vi "Create Plugins.vi"(8 "error in (no error)":errorcluster, 9 "async plugins tag":string, 10 "inline plugins tag":string, 11 "Application Data In":T1={"Item Tree Control"=refnum, "Top-Level VI"=refnum, "menu reference"=refnum, "queue"=refnum, "Stop Pointer"=refnum, "Buffer Variant"=variant, "server ID"=refnum, "framework tag"="", "Values"=refnum, "Hex"=refnum, "ASCII"=refnum, "lines visible"=0, "values padding"=0, "current buffer data"={"decimation"=0, "avg bandwidth"=0.0, "channels"=[], "byte order"=enum."little-endian", "buffer descriptor"={"buffer type"=enum."Engine", "plugin id"=0, "group id"=0, "transfer id"=0, "offset"=0, "length"=0}, "values channels"={"index"=0, "count"=0, "engine offset"=0}, "select start offset"=18446744073709551615, "select end offset"=0, "channel index"=-1}, "Framework Configuration"=refnum} {"current buffer data"."channels"."configuration"."string offset" format="%d bytes"; "current buffer data"."avg bandwidth" format="%.0g bytes"}) -> (0 "error out":errorcluster, 2 "avg bandwidth":dbl, 3 "Application Data out":T1={"Item Tree Control"=refnum, "Top-Level VI"=refnum, "menu reference"=refnum, "queue"=refnum, "Stop Pointer"=refnum, "Buffer Variant"=variant, "server ID"=refnum, "framework tag"="", "Values"=refnum, "Hex"=refnum, "ASCII"=refnum, "lines visible"=0, "values padding"=0, "current buffer data"={"decimation"=0, "avg bandwidth"=0.0, "channels"=[], "byte order"=enum."little-endian", "buffer descriptor"={"buffer type"=enum."Engine", "plugin id"=0, "group id"=0, "transfer id"=0, "offset"=0, "length"=0}, "values channels"={"index"=0, "count"=0, "engine offset"=0}, "select start offset"=18446744073709551615, "select end offset"=0, "channel index"=-1}, "Framework Configuration"=refnum} {"current buffer data"."channels"."configuration"."string offset" format="%d bytes"; "current buffer data"."avg bandwidth" format="%.0g bytes"})   [LabVIEW 2020, in "DSF Core.lvlib"]
uses:
  DSF Core.lvlib
  Buffer Reader/Buffer Data.ctl
  Typedefs/DSF Data Type.ctl
  Typedefs/DSF Byte Order.ctl
  Typedefs/DSF Settings Info.ctl
  Typedefs/DSF Buffer Type.ctl
  Classes/Thread/Data Server/DSF Buffer Subset Descriptor.ctl
  Main VI/Values Channels.ctl
  Typedefs/Core Channel Configuration.ctl
  Classes/Configuration/Core/Channel/Channel Configuration.lvclass
  Classes/Configuration/Core/Framework/Framework Configuration.lvclass
  Classes/Configuration/Core/Plugin/Plugin Configuration.lvclass
  Classes/Configuration/Core/Transfer/Channel Configuration.ctl
  Classes/Configuration/Core/Transfer/Transfer Configuration.lvclass
  Main VI/Application Data.ctl
  <vilib>/NI/Memory Manager/Classes/Pointer/Pointer.lvclass
  Buffer Reader/Queue Data.ctl
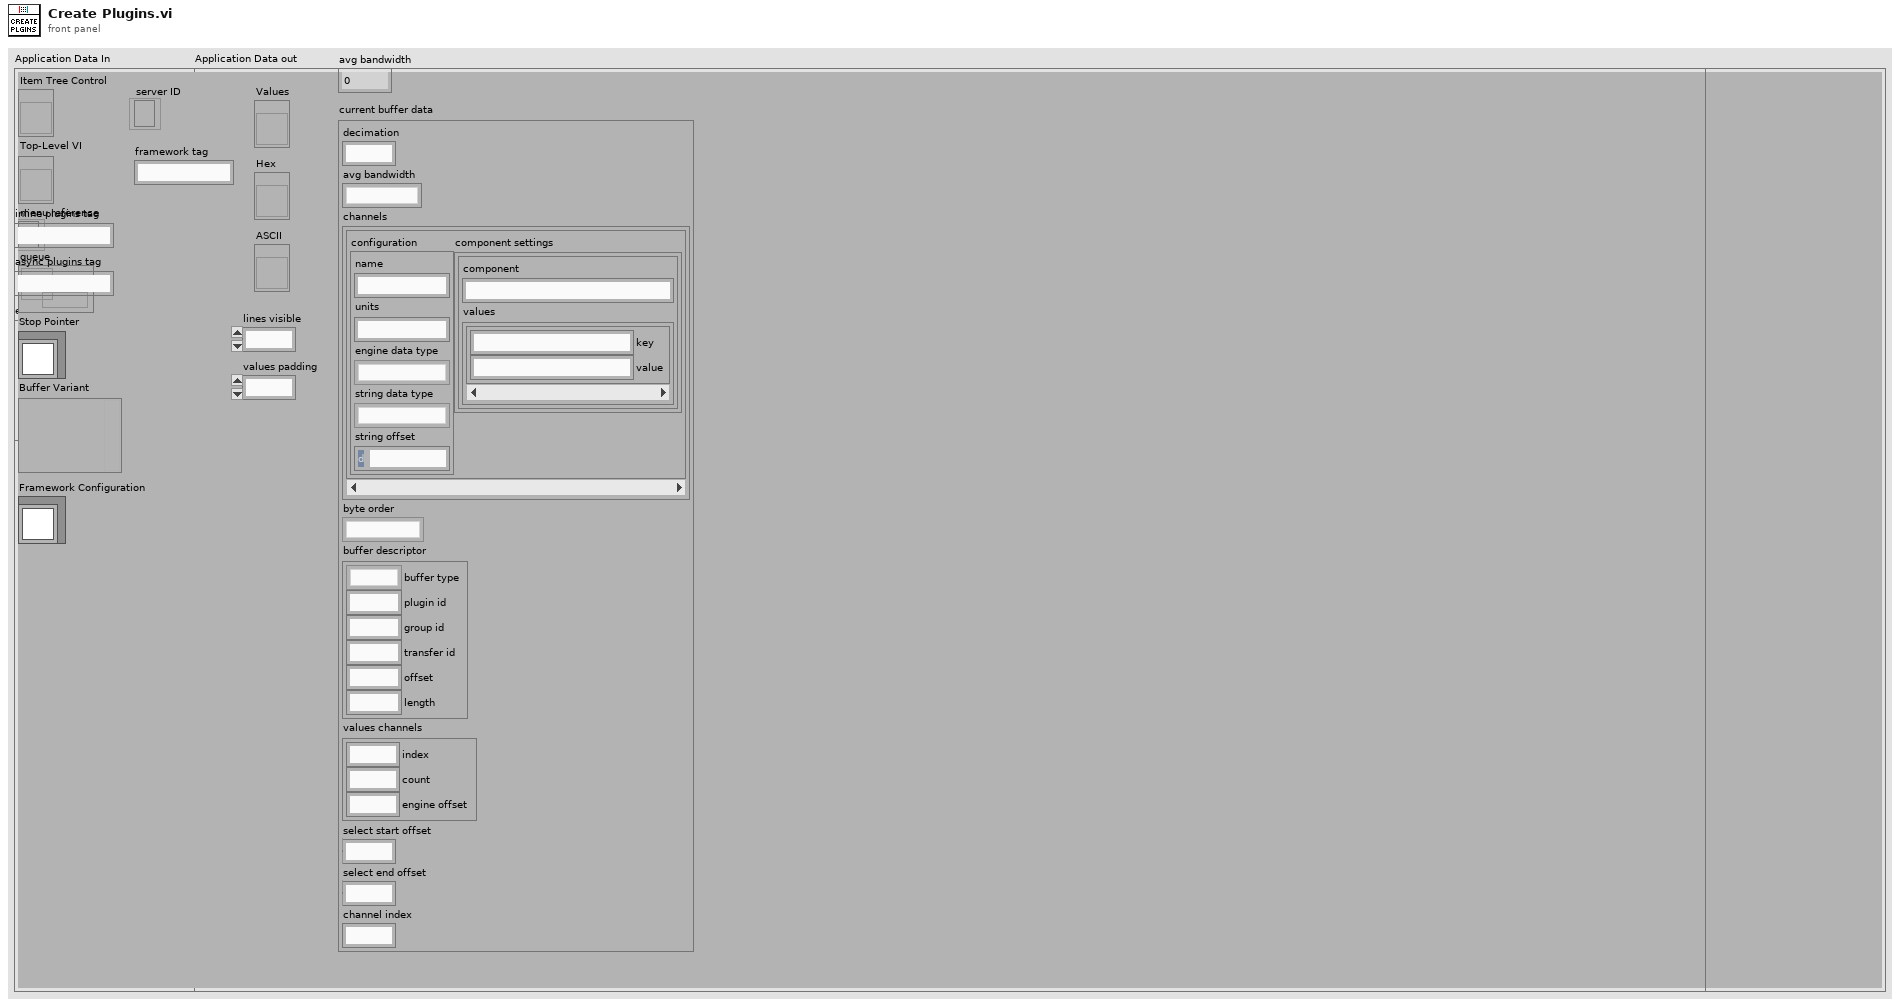
[diagram p1: front panel]
types:
  T1 = typedef "DSF Core.lvlib/Application Data.ctl" = cluster{"Item Tree Control":refnum<vi>, "Top-Level VI":refnum<vi>, "menu reference":refnum<k9>, "queue":refnum<queue>, "Stop Pointer":refnum<class "Pointer.lvclass">, "Buffer Variant":variant, "server ID":refnum<k5>, "framework tag":string, "Values":refnum<vi>, "Hex":refnum<vi>, "ASCII":refnum<vi>, "lines visible":i32, "values padding":i32, "current buffer data":T2, "Framework Configuration":refnum<class "Framework Configuration.lvclass">}
  T2 = typedef "DSF Core.lvlib/Buffer Data.ctl" = cluster{"decimation":u64, "avg bandwidth":dbl, "channels":T3[], "byte order":T7, "buffer descriptor":T8, "values channels":T10, "select start offset":u64, "select end offset":u64, "channel index":i32}
  T3 = typedef "DSF Core.lvlib/Transfer Configuration.lvclass/Channel Configuration.ctl" = cluster{"configuration":T4, "component settings":T6[]}
  T4 = typedef "DSF Core.lvlib/Channel Configuration.lvclass/Core Channel Configuration.ctl" = cluster{"name":string, "units":string, "engine data type":T5, "string data type":T5, "string offset":u64}
  T5 = typedef "DSF Core.lvlib/DSF Data Type.ctl" = enum8{"Bool", "SGL", "DBL", "I8", "I16", "I32", "I64", "U8", "U16", "U32", "U64"}
  T6 = typedef "DSF Core.lvlib/DSF Settings Info.ctl" = cluster{"component":string, "values":cluster{"key":string, "value":string}[]}
  T7 = typedef "DSF Core.lvlib/DSF Byte Order.ctl" = enum8{"big-endian", "little-endian"}
  T8 = typedef "DSF Core.lvlib/DSF Buffer Subset Descriptor.ctl" = cluster{"buffer type":T9, "plugin id":i32, "group id":i32, "transfer id":i32, "offset":u64, "length":i64}
  T9 = typedef "DSF Core.lvlib/DSF Buffer Type.ctl" = enum16{"Engine", "String"}
  T10 = typedef "DSF Core.lvlib/Values Channels.ctl" = cluster{"index":i32, "count":i32, "engine offset":u64}
  T11 = typedef "DSF Core.lvlib/DSF Timing Info.ctl" = cluster{"priority":u64, "decimation":u64, "offset":u64}
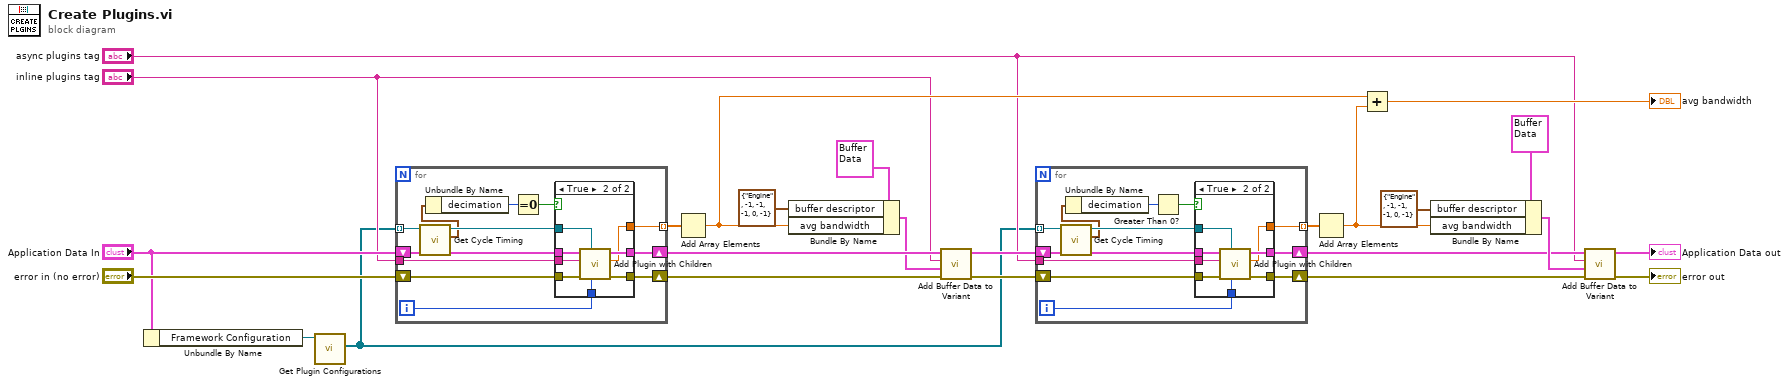
[diagram p0: block diagram]
diagram:
  n1 = Unbundle By Name("Application Data In") -> ("Framework Configuration"=w2:refnum<class "Framework Configuration.lvclass">)
  n2 = call "Get Plugin Configurations.vi"("Framework Configuration in"=w2) -> ("Plugin Configurations"=w1:refnum<class "Plugin Configuration.lvclass">[])  [unwired: 8 in, 2 out]
  n3 = for {
    shift-right: [w34] -> w21
    shift-left: "error in (no error)" -> [w36]
    tunnel: "inline plugins tag" -> [w32]
    shift-right: [w35] -> w22
    shift-left: "Application Data In" -> [w37]
    tunnel: [w33] -> w24 mode=indexing
    tunnel: w1 -> [w28] mode=indexing
    i -> [w31]
    n4 = call "Get Cycle Timing.vi"("Plugin Configuration in"=w28) -> ("cycle timing"=w26:T11, "Plugin Configuration out"=w27:refnum<class "Plugin Configuration.lvclass">)  [unwired: 8 in, 1 out]
    n5 = Unbundle By Name(w26) -> ("decimation"=w30:u64)
    n6 = Equal To 0?(x=w30) -> (x = 0?=w29:bool)
    n7 = case shown="True" w29 {
      tunnel: w37 -> [w39 w47]
      tunnel: w36 -> [w38 w46]
      tunnel: [w39 w45] -> w35
      tunnel: [w38 w44] -> w34
      tunnel: [_ w43] -> w33
      tunnel: w32 -> [_ w42]
      tunnel: w31 -> [_ w41]
      tunnel: w27 -> [_ w40]
      frame False {
      }
      frame True {
        n8 = call "Add Plugin with Children.vi"("ID"=w41, "Plugin Configuration"=w40, "error in (no error)"=w46, "parent tag"=w42, "Application Data In"=w47) -> ("error out"=w44:errorcluster, "average bandwidth"=w43:dbl, "Application Data Out"=w45:T1)  [unwired: 4 in]
      }
    }
  }
  n9 = Add Array Elements(numeric array=w24) -> (sum=w10:dbl)
  n10 = Bundle By Name(cluster=T2 {"decimation"=0, "avg bandwidth"=0.0, "channels"=[], "byte order"=enum."big-endian", "buffer descriptor"={"buffer type"=enum."Engine", "plugin id"=0, "group id"=0, "transfer id"=0, "offset"=0, "length"=0}, "values channels"={"index"=0, "count"=0, "engine offset"=0}, "select start offset"=18446744073709551615, "select end offset"=0, "channel index"=-1} ("Buffer data"), "buffer descriptor"=T8 {"buffer type"=enum."Engine", "plugin id"=-1, "group id"=-1, "transfer id"=-1, "offset"=0, "length"=-1}, "avg bandwidth"=w10) -> (w18:T2)
  n11 = call "Add Buffer Data to Variant.vi"("error in (no error)"=w21, "Buffer data"=w18, "tag"="inline plugins tag", "Application Data In in"=w22) -> ("error out"=w9:errorcluster, "Application Data In out"=w8:T1)  [unwired: 6 in]
  n12 = for {
    shift-right: [w56] -> w5
    shift-left: w9 -> [w58]
    tunnel: "async plugins tag" -> [w54]
    shift-right: [w57] -> w6
    shift-left: w8 -> [w59]
    tunnel: [w55] -> w7 mode=indexing
    tunnel: w1 -> [w50] mode=indexing
    i -> [w53]
    n13 = call "Get Cycle Timing.vi"("Plugin Configuration in"=w50) -> ("cycle timing"=w48:T11, "Plugin Configuration out"=w49:refnum<class "Plugin Configuration.lvclass">)  [unwired: 8 in, 1 out]
    n14 = Unbundle By Name(w48) -> ("decimation"=w52:u64)
    n15 = Greater Than 0?(x=w52) -> (x > 0?=w51:bool)
    n16 = case shown="True" w51 {
      tunnel: w59 -> [w61 w69]
      tunnel: w58 -> [w60 w68]
      tunnel: [w61 w67] -> w57
      tunnel: [w60 w66] -> w56
      tunnel: [_ w65] -> w55
      tunnel: w54 -> [_ w64]
      tunnel: w53 -> [_ w63]
      tunnel: w49 -> [_ w62]
      frame False {
      }
      frame True {
        n17 = call "Add Plugin with Children.vi"("ID"=w63, "Plugin Configuration"=w62, "error in (no error)"=w68, "parent tag"=w64, "Application Data In"=w69) -> ("error out"=w66:errorcluster, "average bandwidth"=w65:dbl, "Application Data Out"=w67:T1)  [unwired: 4 in]
      }
    }
  }
  n18 = Add Array Elements(numeric array=w7) -> (sum=w16:dbl)
  n19 = Add(x=w10, y=w16) -> (x+y=→"avg bandwidth":dbl)
  n20 = Bundle By Name(cluster=T2 {"decimation"=0, "avg bandwidth"=0.0, "channels"=[], "byte order"=enum."big-endian", "buffer descriptor"={"buffer type"=enum."Engine", "plugin id"=0, "group id"=0, "transfer id"=0, "offset"=0, "length"=0}, "values channels"={"index"=0, "count"=0, "engine offset"=0}, "select start offset"=18446744073709551615, "select end offset"=0, "channel index"=-1} ("Buffer data"), "buffer descriptor"=T8 {"buffer type"=enum."Engine", "plugin id"=-1, "group id"=-1, "transfer id"=-1, "offset"=0, "length"=-1}, "avg bandwidth"=w16) -> (w15:T2)
  n21 = call "Add Buffer Data to Variant.vi"("error in (no error)"=w5, "Buffer data"=w15, "tag"="async plugins tag", "Application Data In in"=w6) -> ("error out"=→"error out":errorcluster, "Application Data In out"=→"Application Data out":T1)  [unwired: 6 in]
